vi "ALTS-2015 Task at Station.vi"(6 "Options":T1=enum."Read", 7 "Read Station":T2, 8 "error in (no error)":errorcluster, 10 "Station # Load":T2, 11 "Serial Details in":T3) -> (0 "error out":errorcluster, 2 "Task @ Station":T3, 3 "Tasks @ All Stations":T3[](array[typedef]))   [LabVIEW 2013]
uses:
  Controls/ALTS-2015 Station Cluster.ctl
  Controls/ALTS-2015 Serial Details.ctl
  Controls/ALTS-2015 Robot Tasks.ctl
  Controls/ALTS-2015 Serial DB Details.ctl
  Controls/ALTS-2015 Task at Station Options.ctl
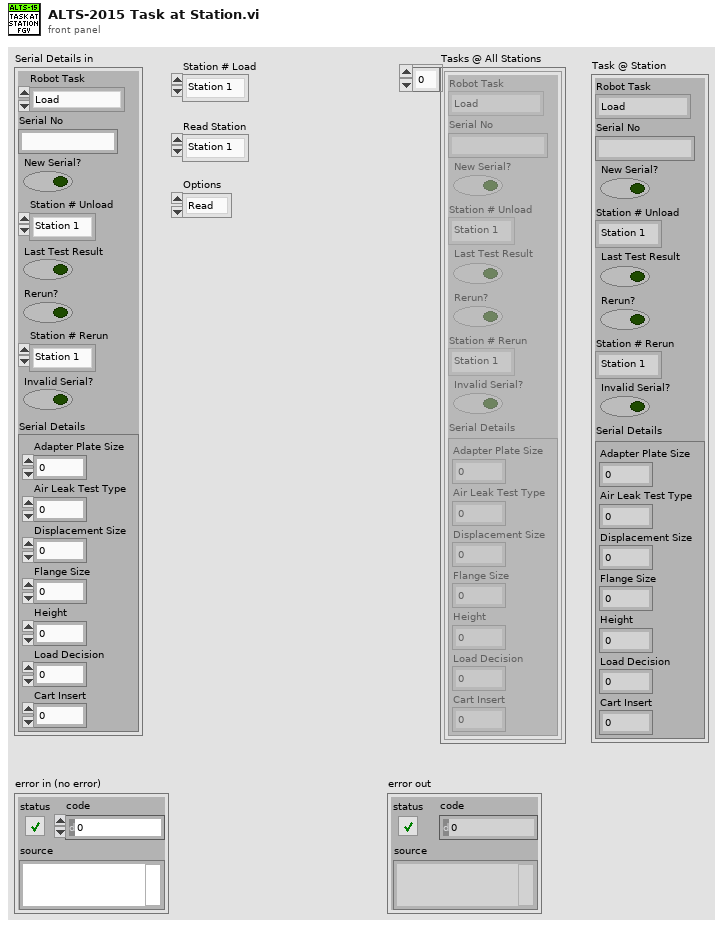
[diagram p1: front panel]
types:
  T1 = typedef "ALTS-2015 Task at Station Options.ctl" = enum16{"Init", "Write", "Read All", "Read"}
  T2 = typedef "ALTS-2015 Station Cluster.ctl" = enum16{"Station 1", "Station 2", "Station 3", "Station 4"}
  T3 = typedef "ALTS-2015 Serial Details.ctl" = cluster{"Robot Task":T4, "Serial No":string, "New Serial?":bool, "Station # Unload":T2, "Last Test Result":bool, "Rerun?":bool, "Station # Rerun":T2, "Invalid Serial?":bool, "Serial Details":T5}
  T4 = typedef "ALTS-2015 Robot Tasks.ctl" = enum16{"Load", "Unload", "Rerun", "Invalid Serial"}
  T5 = typedef "ALTS-2015 Serial DB Details.ctl" = cluster{"Adapter Plate Size":i32, "Air Leak Test Type ":i32, "Displacement Size":i32, "Flange Size":i32, "Height":i32, "Load Decision":i32, "Cart Insert":i32}
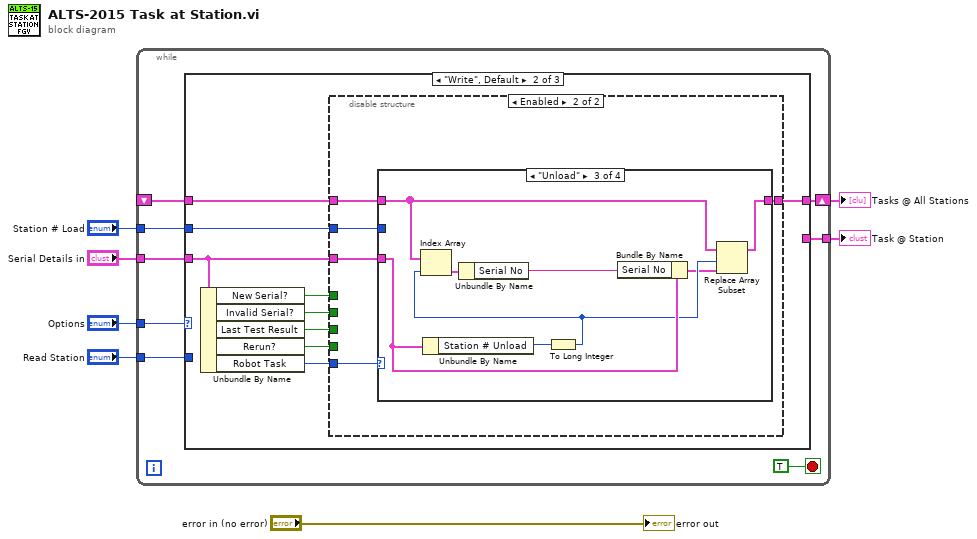
[diagram p0: block diagram]
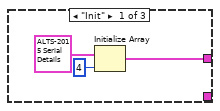
[diagram p2: hidden frame]
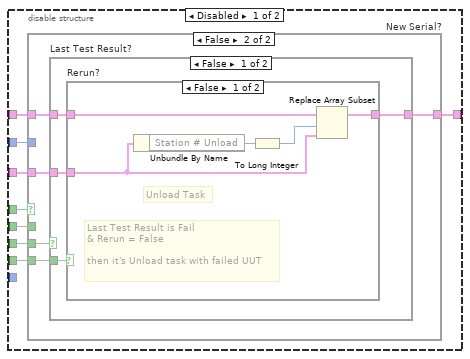
[diagram p3: hidden frame]
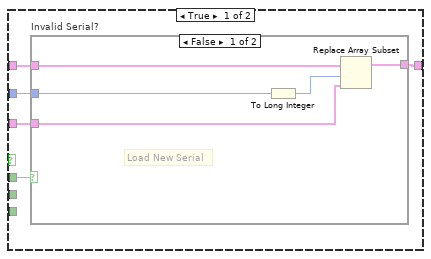
[diagram p4: hidden frame]
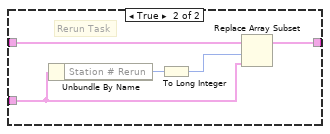
[diagram p6: hidden frame]
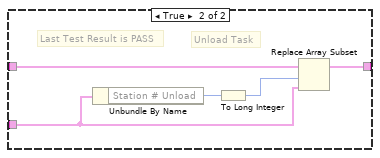
[diagram p7: hidden frame]
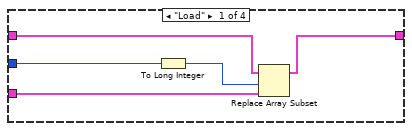
[diagram p8: hidden frame]
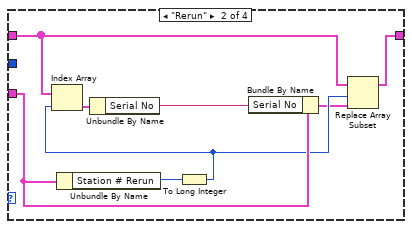
[diagram p9: hidden frame]
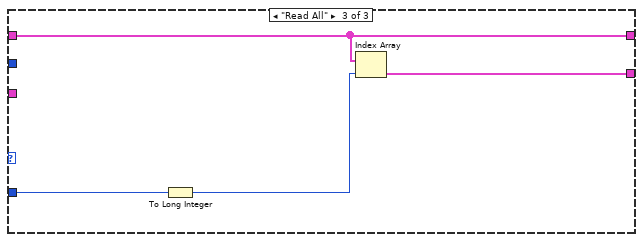
[diagram p11: hidden frame]
diagram:
  n1 = while {
    shift-right: [w14] -> w4
    shift-left: _ -> [w15]
    tunnel: "Station # Load" -> [w13]
    tunnel: "Serial Details in" -> [w12]
    tunnel: "Options" -> [w10]
    tunnel: [w9] -> w3
    tunnel: "Read Station" -> [w8]
    stop <- TRUE stop-if-true
    n2 = case shown="\"Write\", Default" w10 {
      tunnel: w15 -> [_ w21 w101]
      tunnel: [w16 w22 w101] -> w14
      tunnel: w13 -> [_ w23 _]
      tunnel: w12 -> [_ w20 _]
      tunnel: [_ _ w100] -> w9
      tunnel: w8 -> [_ _ w99]
      frame "Init" {
        n3 = Initialize Array(T3 {"Robot Task"=enum."Load", "Serial No"="", "New Serial?"=FALSE, "Station # Unload"=enum."Station 1", "Last Test Result"=FALSE, "Rerun?"=FALSE, "Station # Rerun"=enum."Station 1", "Invalid Serial?"=FALSE, "Serial Details"={"Adapter Plate Size"=0, "Air Leak Test Type "=0, "Displacement Size"=0, "Flange Size"=0, "Height"=0, "Load Decision"=0, "Cart Insert"=0}} ("Serial Details in"), 4 ("dimension size")) -> (w16:T3[])
      }
      frame "Write", Default {
        n4 = Unbundle By Name(w20) -> ("New Serial?"=w27:bool, "Invalid Serial?"=w24:bool, "Last Test Result"=w26:bool, "Rerun?"=w25:bool, "Robot Task"=w19:T4)
        n5 = disable-structure shown="Enabled" {
          disable-tunnel: w27 -> [w35 _]
          disable-tunnel: w26 -> [w34 _]
          disable-tunnel: w25 -> [w33 _]
          disable-tunnel: w24 -> [w32 _]
          disable-tunnel: w23 -> [w31 w71]
          disable-tunnel: [w30 w74] -> w22
          disable-tunnel: w21 -> [w29 w75]
          disable-tunnel: w20 -> [w28 w72]
          disable-tunnel: w19 -> [_ w73]
          frame Disabled {
            n6 = case "New Serial?" shown="False" w35 {
              tunnel: w34 -> [_ w51]
              tunnel: w33 -> [_ w50]
              tunnel: w32 -> [w40 _]
              tunnel: w31 -> [w39 _]
              tunnel: [w38 w49] -> w30
              tunnel: w29 -> [w37 w48]
              tunnel: w28 -> [w36 w47]
              frame True {
                n7 = case "Invalid Serial?" shown="False" w40 {
                  tunnel: w39 -> [w42 _]
                  tunnel: [w44 w46] -> w38
                  tunnel: w37 -> [w43 w46]
                  tunnel: w36 -> [w41 _]
                  frame False {
                    # "Load New Serial"
                    n8 = To Long Integer(number=w42) -> (32bit integer=w45:i32)
                    n9 = Replace Array Subset(array=w43, new element=w41, index=w45) -> (w44:T3[])
                  }
                  frame True {
                    # "Don't update if Invalid.  Invalid serials\nwill not go to any stations."
                  }
                }
              }
              frame False {
                n10 = case "Last Test Result?" shown="False" w51 {
                  tunnel: w50 -> [w55 _]
                  tunnel: [w54 w68] -> w49
                  tunnel: w48 -> [w53 w69]
                  tunnel: w47 -> [w52 w67]
                  frame False {
                    n11 = case "Rerun?" shown="False" w55 {
                      tunnel: [w58 w63] -> w54
                      tunnel: w53 -> [w59 w64]
                      tunnel: w52 -> [w56 w61]
                      frame False {
                        # "Unload Task"
                        # "Last Test Result is Fail\n& Rerun = False\n\nthen it's Unload task with failed UUT"
                        n12 = Unbundle By Name(w56) -> ("Station # Unload"=w57:T2)
                        n13 = To Long Integer(number=w57) -> (32bit integer=w60:i32)
                        n14 = Replace Array Subset(array=w59, new element=w56, index=w60) -> (w58:T3[])
                      }
                      frame True {
                        # "Rerun Task"
                        n15 = Unbundle By Name(w61) -> ("Station # Rerun"=w62:T2)
                        n16 = To Long Integer(number=w62) -> (32bit integer=w65:i32)
                        n17 = Replace Array Subset(array=w64, new element=w61, index=w65) -> (w63:T3[])
                      }
                    }
                  }
                  frame True {
                    # "Unload Task"
                    # "Last Test Result is PASS"
                    n18 = Unbundle By Name(w67) -> ("Station # Unload"=w66:T2)
                    n19 = To Long Integer(number=w66) -> (32bit integer=w70:i32)
                    n20 = Replace Array Subset(array=w69, new element=w67, index=w70) -> (w68:T3[])
                  }
                }
              }
            }
          }
          frame Enabled {
            n21 = case shown="\"Unload\"" w73 {
              tunnel: w75 -> [w80 w85 w93 w97]
              tunnel: [w79 w88 w96 w97] -> w74
              tunnel: w72 -> [w77 w86 w94 _]
              tunnel: w71 -> [w76 _ _ _]
              frame "Load" {
                n22 = To Long Integer(number=w76) -> (32bit integer=w78:i32)
                n23 = Replace Array Subset(array=w80, new element=w77, index=w78) -> (w79:T3[])
              }
              frame "Rerun" {
                n24 = Unbundle By Name(w86) -> ("Station # Rerun"=w87:T2)
                n25 = To Long Integer(number=w87) -> (32bit integer=w84:i32)
                n26 = Index Array(array=w85, index=w84) -> (element=w83:T3)
                n27 = Unbundle By Name(w83) -> ("Serial No"=w81:string)
                n28 = Bundle By Name(cluster=w86, "Serial No"=w81) -> (w82:T3)
                n29 = Replace Array Subset(array=w85, new element=w82, index=w84) -> (w88:T3[])
              }
              frame "Unload" {
                n30 = Unbundle By Name(w94) -> ("Station # Unload"=w95:T2)
                n31 = To Long Integer(number=w95) -> (32bit integer=w92:i32)
                n32 = Index Array(array=w93, index=w92) -> (element=w91:T3)
                n33 = Unbundle By Name(w91) -> ("Serial No"=w89:string)
                n34 = Bundle By Name(cluster=w94, "Serial No"=w89) -> (w90:T3)
                n35 = Replace Array Subset(array=w93, new element=w90, index=w92) -> (w96:T3[])
              }
              frame "Invalid Serial" {
              }
            }
          }
        }
      }
      frame "Read All" {
        n36 = To Long Integer(number=w99) -> (32bit integer=w98:i32)
        n37 = Index Array(array=w101, index=w98) -> (element=w100:T3)
      }
    }
  }
  "Tasks @ All Stations" <- w4
  "Task @ Station" <- w3
  "error out" <- "error in (no error)"
